vi "Read point-to-point.vi"(1 "Worksheet Name":string="PXI-6238", 2 "Path":path=path "X:/Lab Configuration/point-to-point.xlsx") -> (0 "Array Out":string[][](array[string]))   [LabVIEW 2018]
doc: "Demonstrates how to use the LabVIEW Report Generator Toolkit to read information from an Excel file\n\nIf you want to know which Excel version is compatible with a certain Report Generation Toolkit see:\n\nKB 3EJEC9NS: Report Generation Toolkit Compatibility with Microsoft Office and LabVIEW\nhttp://digital.ni.com/public.nsf/allkb/C9408B9F08D711E786256F3300701D01"
uses:
  <vilib>/Utility/NIReport.llb/Report Type.ctl
  <vilib>/addons/_office/excel.llb/Excel Get Data ([str]).vi
  <vilib>/Utility/NIReport.llb/NI_report.lvclass
  <vilib>/Utility/NIReport.llb/Excel/NI_Excel.lvclass
  <vilib>/addons/_office/NI_ReportGenerationToolkit.lvlib
  <vilib>/Utility/NIReport.llb/NI_ReportGenerationCore.lvlib
panel:
  in  "Remove rows":i32=2
  # "Overview: Demonstrates how to use the LabVIEW Report Generator Toolkit to read information from an Excel file\nRequirements: LabVIEW 2012 Base Development System (or compatible)\n                             LabVIEW 2012 Report Generation Toolkit (or compatible)\n                             Microsoft Excel\n                             (KB 3EJEC9NS: Report Generation Toolkit Compatibility with Microsoft Office and LabVIEW\n                             http://digital.ni.com/public.nsf/allkb/C9408B9F08D711E786256F3300701D01)\nInstructions: \n1. Run the VI"
  # "Sheet 3"
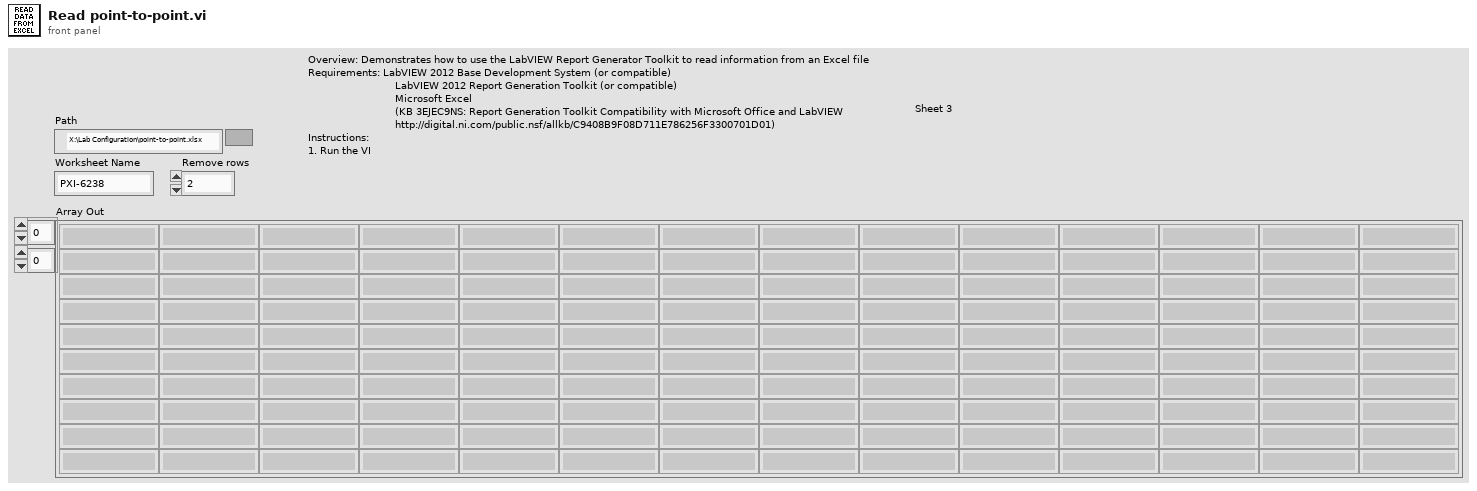
[diagram p1: front panel]
types:
  T1 = typedef "NI_ReportGenerationCore.lvlib/Report Type.ctl" = enum16{"HTML", "Word", "Excel"}
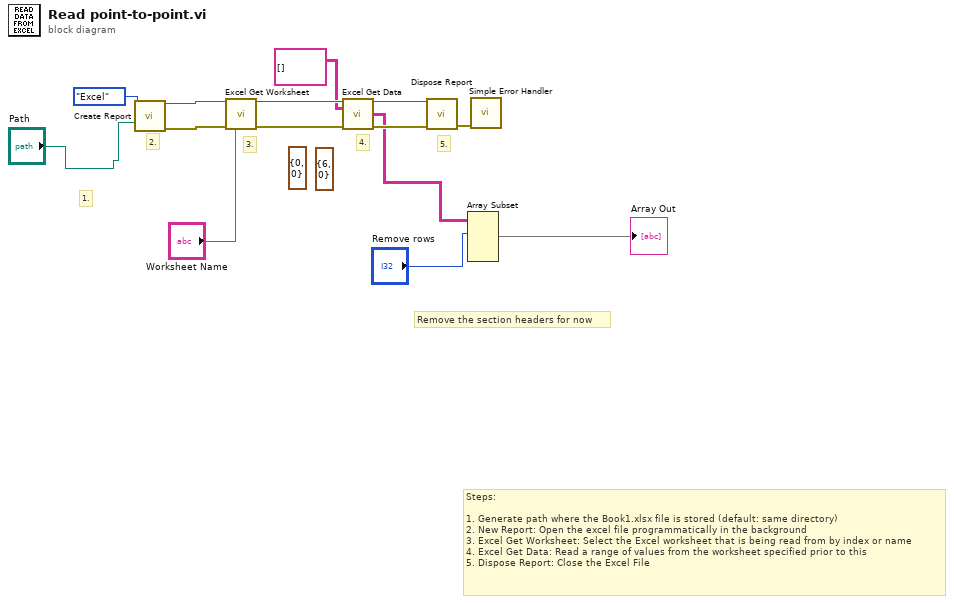
[diagram p0: block diagram]
diagram:
  (unwired) cluster{"row":i32, "column":i32} {"row"=6, "column"=0} ("end (-1, -1)")
  (unwired) cluster{"row":i32, "column":i32} {"row"=0, "column"=0} ("start (-1, -1)")
  # "Remove the section headers for now"
  # "5."
  # "4."
  # "3."
  # "2."
  # "1."
  # "Steps:\n\n1. Generate path where the Book1.xlsx file is stored (default: same directory)\n2. New Report: Open the excel file programmatically in the background\n3. Excel Get Worksheet: Select the Excel worksheet that is being read from by index or name\n4. Excel Get Data: Read a range of values from the worksheet specified prior to this\n5. Dispose Report: Close the Excel File"
  n1 = call <vilib>:"Create Report.vi"("report type"=Report_Type."Excel", "template (empty)"="Path") -> ("report out"=w13:refnum<class "NI_report.lvclass">, "error out"=w14:errorcluster)  [unwired: 12 in]
  n2 = call <vilib>:"Excel Get Worksheet.vi"("report in"=w13, "error in (no error)"=w14, "name (\"\")"="Worksheet Name") -> ("report out"=w10:refnum<class "NI_report.lvclass">, "error out"=w11:errorcluster)  [unwired: 1 in, 10 out]
  n3 = call-poly <vilib>:"Excel Get Data.vi"("report in"=w10, "data type"=string[][] [], "error in (no error)"=w11) -> ("report out"=w7:refnum<class "NI_report.lvclass">, "data"=w3:string[][], "error out"=w8:errorcluster)  [unwired: 10 in]
  n4 = call-dynamic "Dispose Report.vi"("report in"=w7, "error in (no error)"=w8) -> ("error out"=w12:errorcluster)  [unwired: 3 in, 10 out]
  n5 = Array Subset(array=w3, index (row)="Remove rows") -> (→"Array Out":string[][])  [unwired: 3 in]
  n6 = call <vilib>:"Simple Error Handler.vi"("error in (no error)"=w12) -> ()  [unwired: 1 in, 8 out]
